vi "Get Output DMA Refs.vi"(8 "error in (no error)":errorcluster, 10 "Item GUID":string, 11 "Section Ref in":T1 format="%.0x") -> (0 "error out":errorcluster, 1 "Refs":T2(array[cluster]) {"VS Refs" format="%.0x"}, 2 "DMA":T3[](array[typedef]) {"Data Type" format="%.0x"; "DMA.Settings"."DMA Host Buffer" items=["1 Second"=1, "2 Seconds"=2, "5 Seconds"=5, "10 Seconds"=10]; "DMA.Settings"."dt" format="%#_p"; "DMA.Settings"."Update Rate" items=["1 Hz"=1, "2 Hz"=2, "5 Hz"=5, "10 Hz"=10]}, 3 "Section Ref out":T1 format="%.0x")   [LabVIEW 2019, in "FPGA Addon System Explorer.lvlib"]
uses:
  FPGA Addon System Explorer.lvlib
  <vilib>/NI VeriStand/Custom Device API/Custom Device Item Ref.ctl
  Shared/Compiled.DMASettings.ctl
  Shared/Data Type.ctl
  Shared/DMA Settings.ctl
  Shared/Delacing Scheme.ctl
  Shared/DMA Acquisition Mode.ctl
  <vilib>/NI VeriStand/Custom Device API/Waveform Data Reference.ctl
  Shared/FG Action.ctl
  Shared/Constants.vi
  <vilib>/NI VeriStand/Custom Device Tools/Custom Device Utility Library/NI VeriStand - Search for Item by GUID.vi
  <vilib>/NI VeriStand/Custom Device API/Get Item Property (Variant).vi
  <vilib>/NI VeriStand/Custom Device API/NI VeriStand - Set Item Property.vi
  <vilib>/NI VeriStand/Custom Device API/Set Item Property (Variant).vi
  <vilib>/NI VeriStand/Custom Device API/Get Item Property (String).vi
  <vilib>/NI VeriStand/Custom Device API/Get Item Property (U32).vi
  <vilib>/NI VeriStand/Custom Device API/Get Item Property (Double).vi
  <vilib>/NI VeriStand/Custom Device API/Set Item Property (U32).vi
  <vilib>/NI VeriStand/Custom Device API/Set Item Property (Double).vi
  <vilib>/NI VeriStand/Custom Device Tools/Custom Device Utility Library/NI VeriStand - Search for All Items by GUID.vi
  <vilib>/NI VeriStand/Custom Device API/Get Item Property (Dependent Node Pointer).vi
  Shared/FPGA Addon Shared.lvlib
  <vilib>/NI VeriStand/Custom Device API/Custom Device API.lvlib
  <vilib>/NI VeriStand/Custom Device Tools/Custom Device Utility Library/Custom Device Utility Library.lvlib
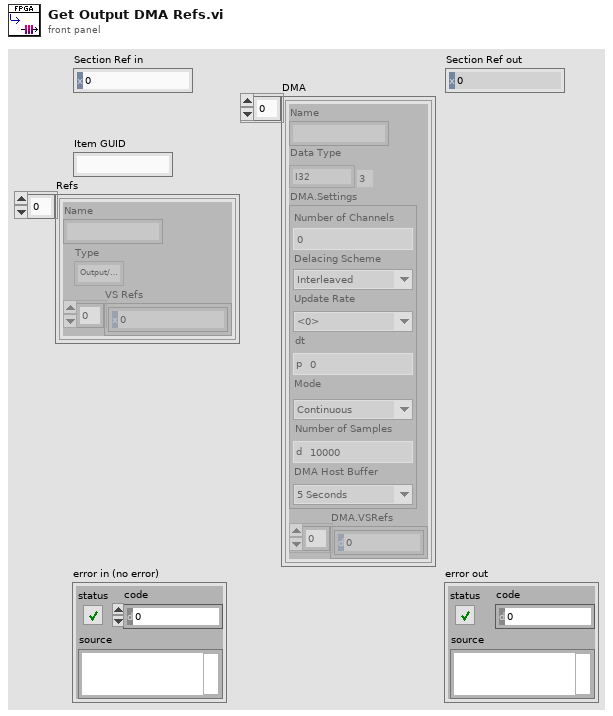
[diagram p1: front panel]
types:
  T1 = typedef "Custom Device API.lvlib/Custom Device Item Ref.ctl" = u64
  T2 = cluster{"Name":string, "Type":enum16{"Output/Write", "Input/Read", "Input/ReadWrite"}, "VS Refs":T1[]}[]
  T3 = typedef "FPGA Addon Shared.lvlib/Compiled.DMASettings.ctl" = cluster{"Name":string, "Data Type":T4, "DMA.Settings":T5, "DMA.VSRefs":T8[]}
  T4 = typedef "FPGA Addon Shared.lvlib/Data Type.ctl" = enum8{"<Null>", "I8", "I16", "I32", "I64", "U8", "U16", "U32", "U64", "SGL", "Boolean", "Analog PWM In Settings", "Analog PWM In", "Digital PWM In Settings", "Digital PWM In", "Digital PWM Out", "Sine Out", "FXP+/-24.5", "FXP+/-16.5", "FXP+/-32.8", "FXP+/-64.32", "FXP+/-16.7", "FXP+/-20.5", "FXP+/-27.5", "FXP+/-32.16", "FXP +16.3", "FXP +18.3", "Digital Static In", "Digital Static Out", "Digital Static In Settings", "Digital WSS Out", "Quad Encoder Settings", "Quad Encoder In"}
  T5 = typedef "FPGA Addon Shared.lvlib/DMA Settings.ctl" = cluster{"Number of Channels":u8, "Delacing Scheme":T6, "Update Rate":u32, "dt":dbl, "Mode":T7, "Number of Samples":u32, "DMA Host Buffer":u32}
  T6 = typedef "FPGA Addon Shared.lvlib/Delacing Scheme.ctl" = enum8{"Interleaved", "Bitpacked"}
  T7 = typedef "FPGA Addon Shared.lvlib/DMA Acquisition Mode.ctl" = enum8{"Continuous", "Triggered Finite"}
  T8 = typedef "Custom Device API.lvlib/Waveform Data Reference.ctl" = i32
  T9 = typedef "FPGA Addon Shared.lvlib/FG Action.ctl" = enum8{"GET", "SET"}
  T10 = typedef "FPGA Addon Shared.lvlib/DMA Information.ctl" = cluster{"Name":string, "Data Type":T4}
  T11 = cluster{"Name":string, "Type":enum16{"Output/Write", "Input/Read", "Input/ReadWrite"}, "VS Refs":T1[]}
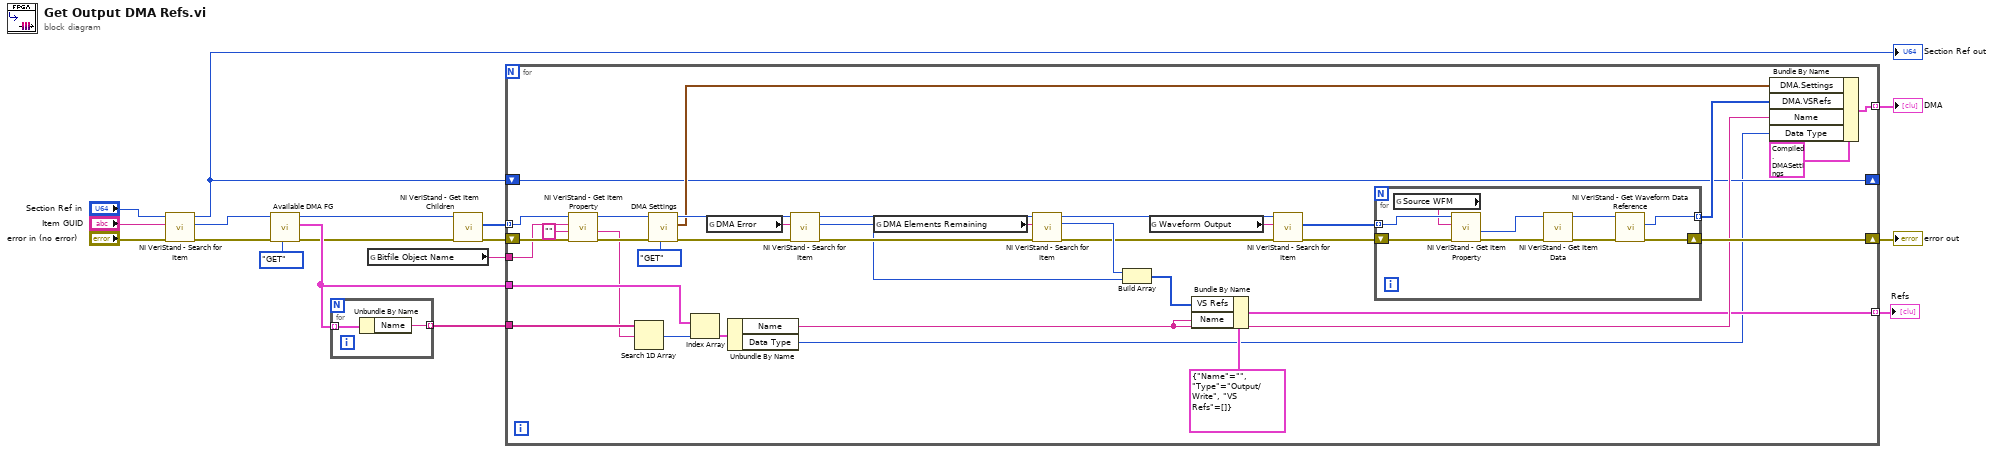
[diagram p0: block diagram]
diagram:
  n1 = call-poly <vilib>:"NI VeriStand - Search for Item.vi"("error in"="error in (no error)", "Item GUID"="Item GUID", "Section Ref in"="Section Ref in") -> ("error out"=w14:errorcluster, "Item Ref"=w16:T1, "Section Ref out"=w3:T1)  [unwired: 5 in, 1 out]
  "Section Ref out" <- w3
  n2 = call "Available DMA FG.vi"("Action"=FG_Action."GET", "error in (no error)"=w14, "Item Ref"=w16) -> ("error out"=w10:errorcluster, "Available DMA"=w11:T10[], "Item Ref out"=w12:T1)  [unwired: 6 in]
  n3 = for {
    tunnel: w11 -> [w19] mode=indexing
    tunnel: [w18] -> w9 mode=indexing
    n4 = Unbundle By Name(w19) -> ("Name"=w18:string)
  }
  n5 = global read "Constants.vi" "Bitfile Object Name"() -> (w8:string)
  n6 = call <vilib>:"NI VeriStand - Get Item Children.vi"("error in (no error)"=w10, "Item Ref in"=w12) -> ("error out"=w6:errorcluster, "Child Refs"=w7:T1[])  [unwired: 6 in, 2 out]
  n7 = for {
    shift-right: [w28] -> w4
    shift-left: w6 -> [w55]
    tunnel: w7 -> [w54] mode=indexing
    tunnel: w8 -> [w53]
    tunnel: w9 -> [w51]
    tunnel: w11 -> [w50]
    tunnel: [w45] -> w2 mode=indexing
    shift-right: [w21] -> _
    shift-left: w3 -> [w21]
    tunnel: [w23] -> w1 mode=indexing
    n8 = call-poly <vilib>:"NI VeriStand - Get Item Property.vi"("error in (no error)"=w55, "Default Value"="", "Property Name"=w53, "Item Ref in"=w54) -> ("error out"=w44:errorcluster, "Value"=w40:string, "Item Ref out"=w43:T1)  [unwired: 4 in, 1 out]
    n9 = Search 1D Array(1D array=w51, element=w40) -> (index of element=w49:i32)  [unwired: 1 in]
    n10 = call "DMA Settings.vi"("Action"=FG_Action."GET", "error in (no error)"=w44, "Item Ref"=w43) -> ("error out"=w38:errorcluster, "DMA Settings"=w30:T5, "Item Ref out"=w37:T1)  [unwired: 6 in]
    n11 = Index Array(array=w50, index=w49) -> (element=w47:T10)
    n12 = global read "Constants.vi" "DMA Error"() -> (w39:string)
    n13 = Unbundle By Name(w47) -> ("Name"=w24:string, "Data Type"=w20:T4)
    n14 = call-poly <vilib>:"NI VeriStand - Search for Item.vi"("error in"=w38, "Item GUID"=w39, "Section Ref in"=w37) -> ("error out"=w35:errorcluster, "Item Ref"=w33:T1, "Section Ref out"=w34:T1)  [unwired: 5 in, 1 out]
    n15 = global read "Constants.vi" "DMA Elements Remaining"() -> (w36:string)
    n16 = call-poly <vilib>:"NI VeriStand - Search for Item.vi"("error in"=w35, "Item GUID"=w36, "Section Ref in"=w34) -> ("error out"=w22:errorcluster, "Item Ref"=w32:T1, "Section Ref out"=w31:T1)  [unwired: 5 in, 1 out]
    n17 = Build Array(w32, w33) -> (w25:T1[])
    n18 = global read "Constants.vi" "Waveform Output"() -> (w41:string)
    n19 = Bundle By Name(cluster=T11 {"Name"="", "Type"=enum."Output/Write", "VS Refs"=[]} ("Group"), "VS Refs"=w25, "Name"=w24) -> (w23:T11)
    n20 = call-poly <vilib>:"NI VeriStand - Search for Item.vi"("error in"=w22, "Item GUID"=w41, "Section Ref in"=w31) -> ("error out"=w42:errorcluster, "Item Refs"=w29:T1[])  [unwired: 5 in, 2 out]
    n21 = for {
      shift-right: [w56] -> w28
      shift-left: w42 -> [w64]
      tunnel: [w57] -> w27 mode=indexing
      tunnel: w29 -> [w63] mode=indexing
      n22 = global read "Constants.vi" "Source WFM"() -> (w62:string)
      n23 = call-poly <vilib>:"NI VeriStand - Get Item Property.vi"("error in (no error)"=w64, "Property Name"=w62, "Item Ref in"=w63) -> ("error out"=w61:errorcluster, "Dependent Node Ref"=w59:T1)  [unwired: 5 in, 2 out]
      n24 = call <vilib>:"NI VeriStand - Get Item Data.vi"("error in (no error)"=w61, "Item Ref in"=w59) -> ("error out"=w60:errorcluster, "Item Ref out"=w58:T1)  [unwired: 8 out]
      n25 = call <vilib>:"NI VeriStand - Get Waveform Data Reference.vi"("error in (no error)"=w60, "Waveform Ref in"=w58) -> ("error out"=w56:errorcluster, "Waveform Data Reference"=w57:T8)  [unwired: 7 in, 1 out]
    }
    n26 = Bundle By Name(cluster=T3 {"Name"="", "Data Type"=enum."I32", "DMA.Settings"={"Number of Channels"=0, "Delacing Scheme"=enum."Interleaved", "Update Rate"=0, "dt"=0.0, "Mode"=enum."Continuous", "Number of Samples"=10000, "DMA Host Buffer"=5}, "DMA.VSRefs"=[]}, "DMA.Settings"=w30, "DMA.VSRefs"=w27, "Name"=w24, "Data Type"=w20) -> (w45:T3)
  }
  "error out" <- w4
  "DMA" <- w2
  "Refs" <- w1
